vi "MTWIPbyPackage.vi"() -> ()   [LabVIEW 2012]
uses:
  <vilib>/Utility/NIReport.llb/NI_report.lvclass
  <vilib>/addons/database/Connection.llb/DB Tools Open Connec (Path).vi
  <vilib>/addons/database/Connection.llb/Conn Execute.vi
  <vilib>/addons/database/Recordset.llb/Rec Fetch Recordset Data (R).vi
  <vilib>/addons/database/Recordset.llb/Rec Destroy - Connection.vi
  <vilib>/Utility/NIReport.llb/Append Text Table to Report (wrap).vi
  <vilib>/addons/database/_DB Variant To Data/Database Variant To Data.xnode
  <vilib>/addons/database/NI_Database_API.lvlib
  <vilib>/Utility/NIReport.llb/Excel/NI_Excel.lvclass
  <vilib>/addons/_office/NI_ReportGenerationToolkit.lvlib
panel:
  out "recordset data 2":variant[][](array[variant])
  out "appended array 2":string[](array[string])
  out "error out 5":errorcluster
  in  "Report Template":path=path "O:/Monitor/Report/M100DailyWIP.xls"
  out "error out 2":errorcluster
  in  "Table Control":string[][](table)
  in  "Table Control 2":string[][](table)
  in  "Table Control 3":string[][](table)
  out "error out 4":errorcluster
  out "error out 3":errorcluster
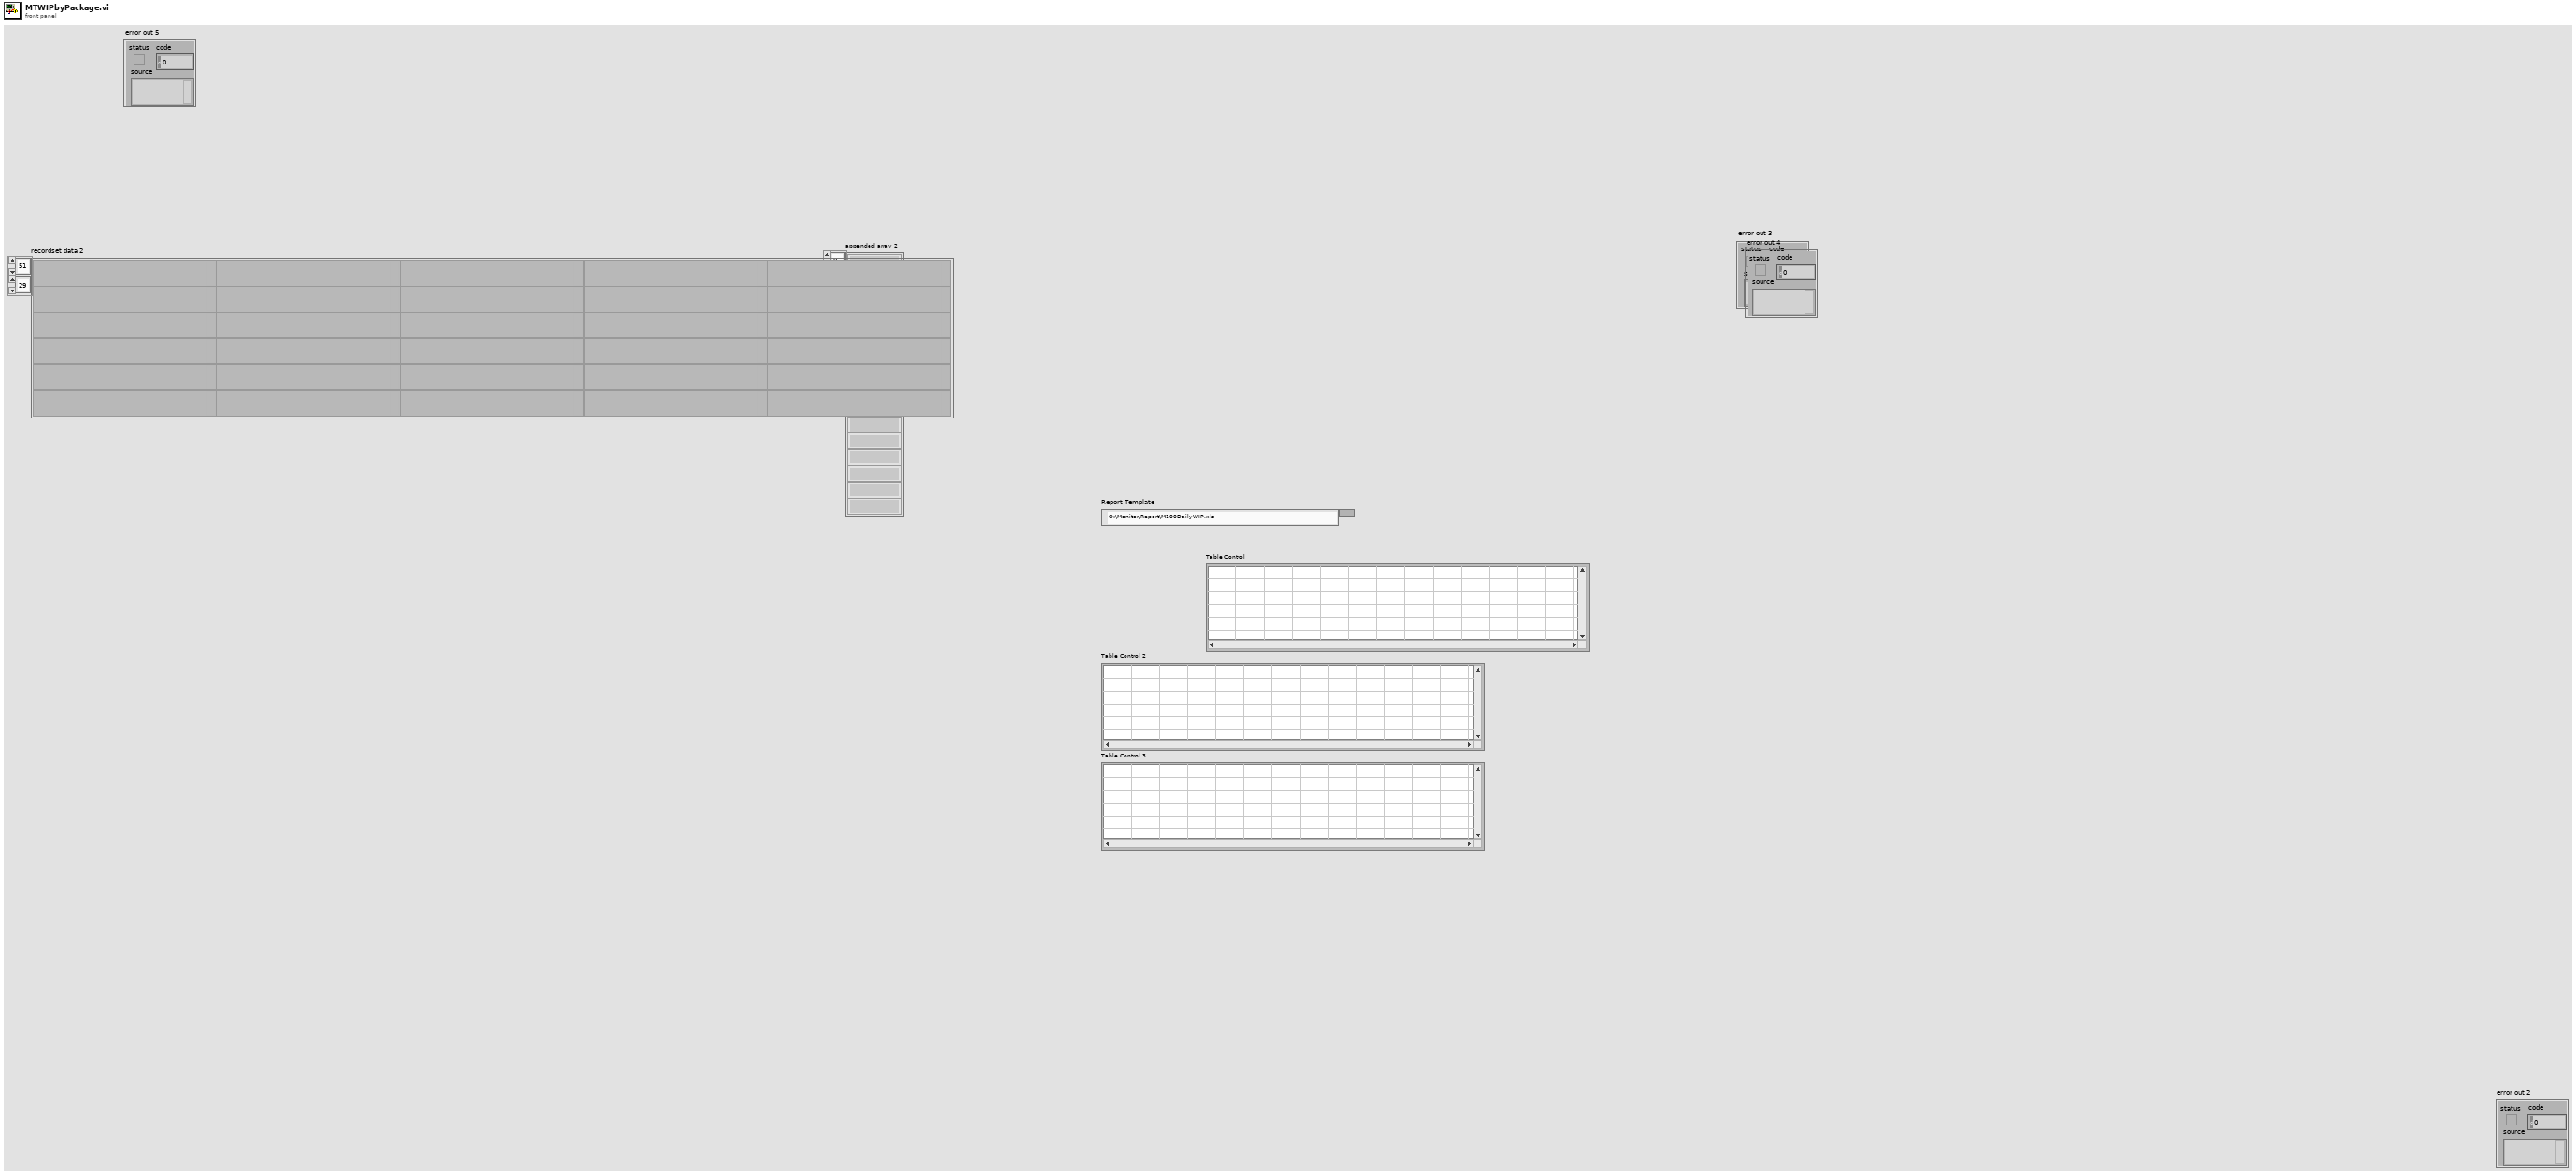
[diagram p1: front panel]
types:
  T1 = typedef "NI_Database_API.lvlib/Conn ObjectReference.ctl" = refnum<k1>
  T2 = typedef "NI_Database_API.lvlib/Rec ObjectReference.ctl" = refnum<k1>
  T3 = enum16{"Standard Report", "HTML", "Word", "Excel"}
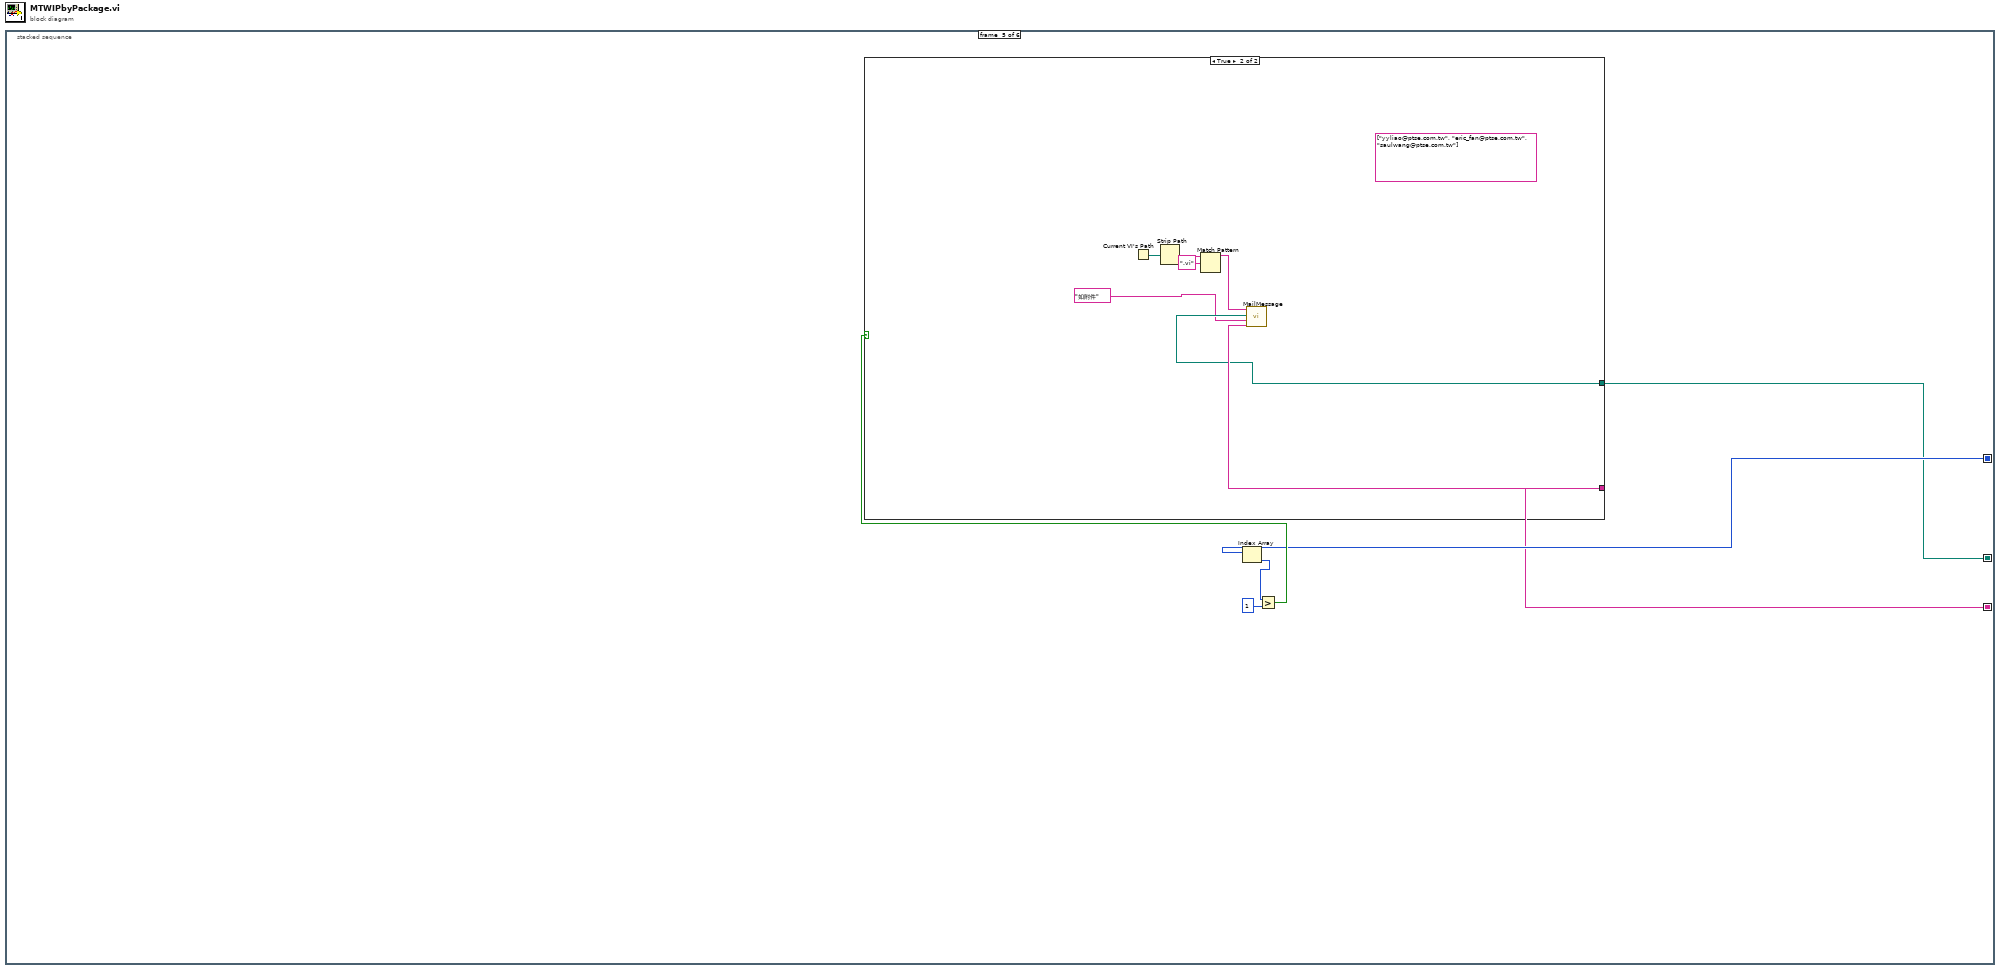
[diagram p0: block diagram]
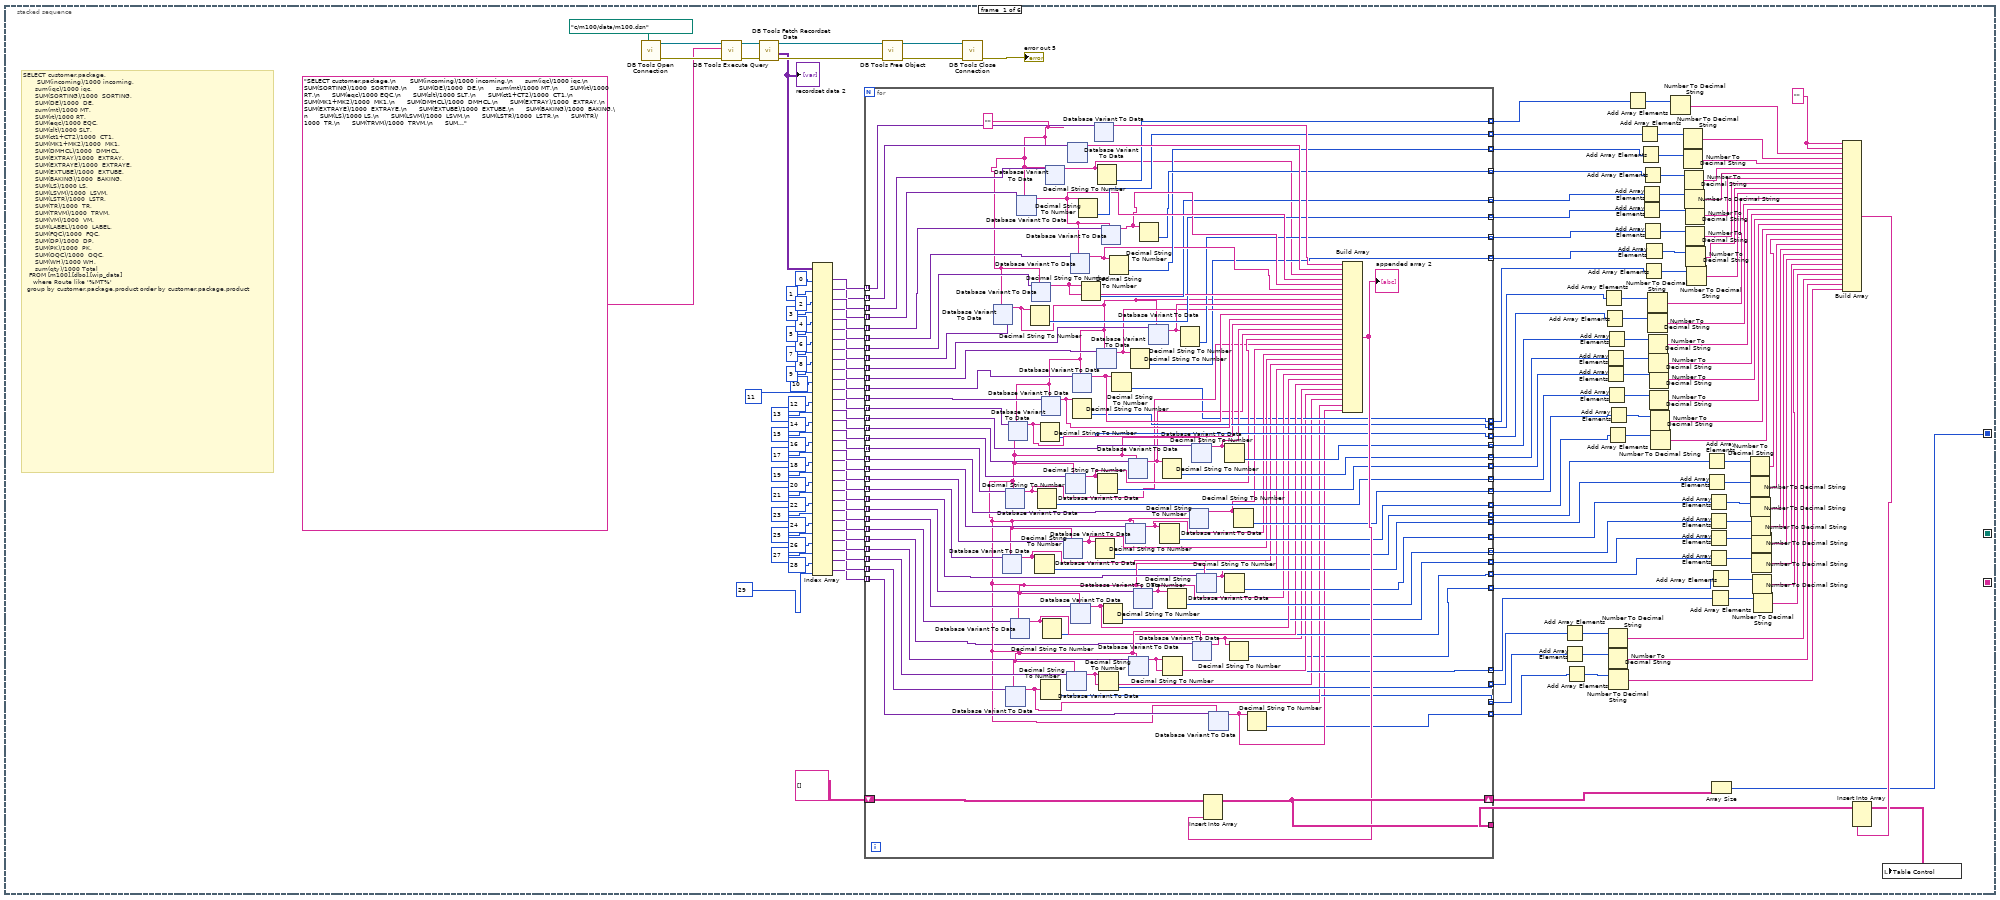
[diagram p2: hidden frame]
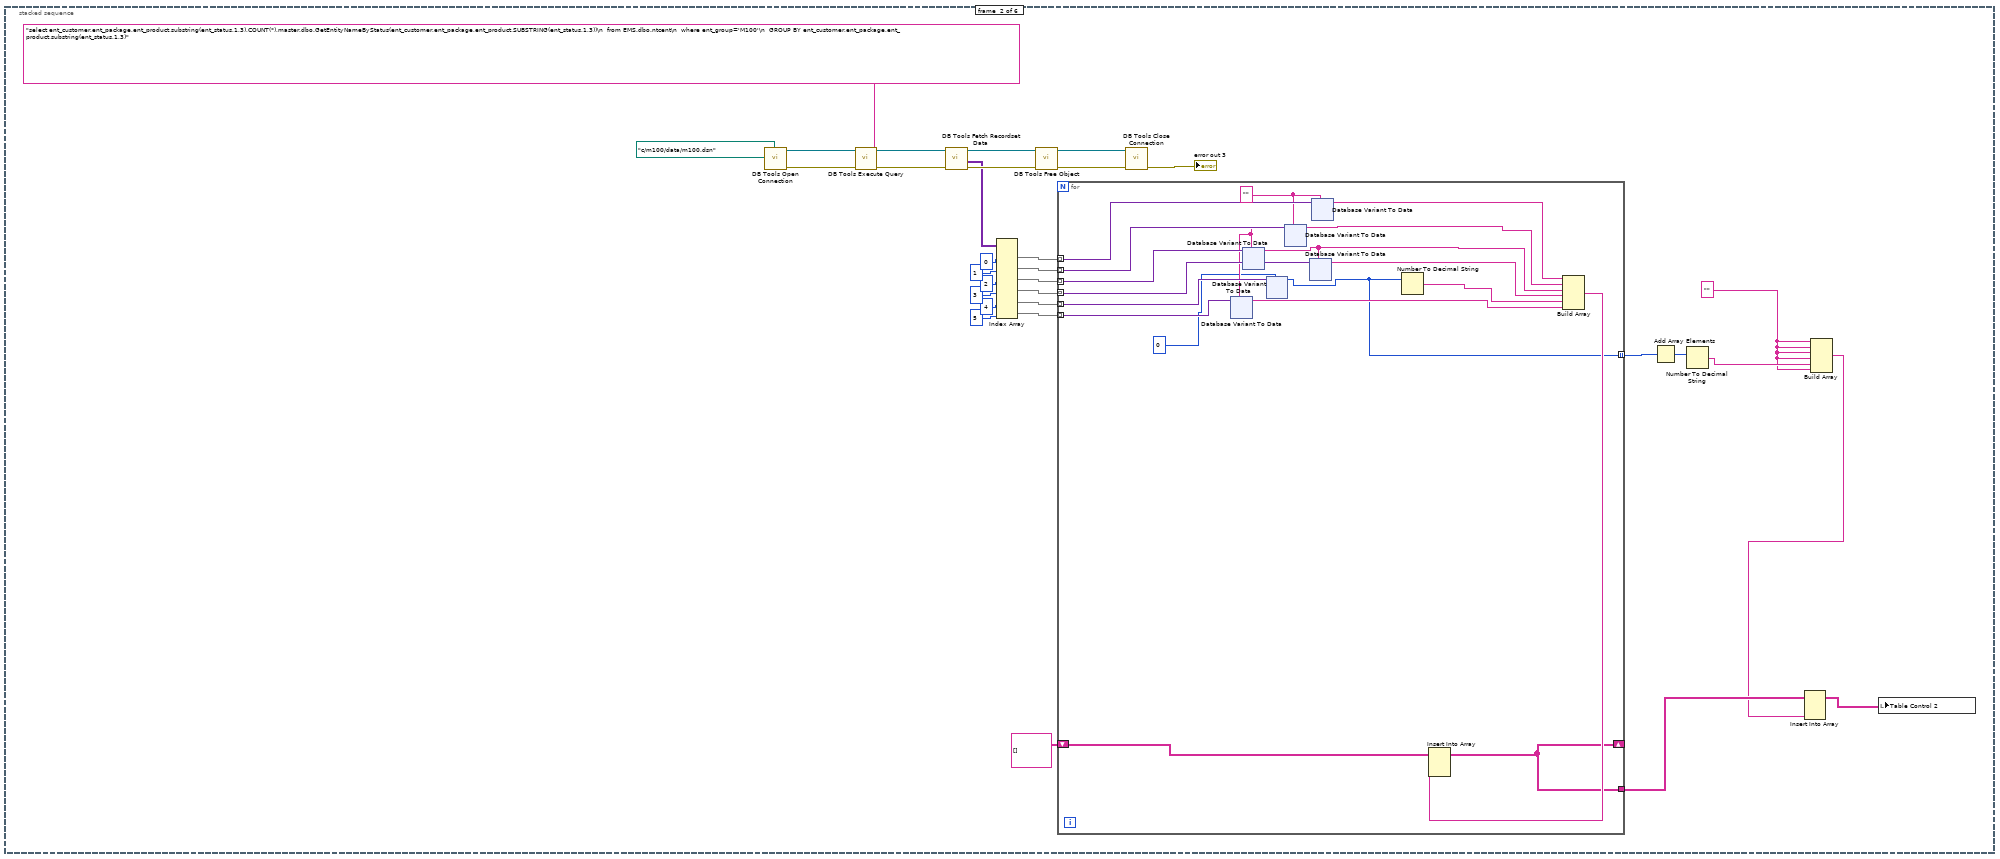
[diagram p3: hidden frame]
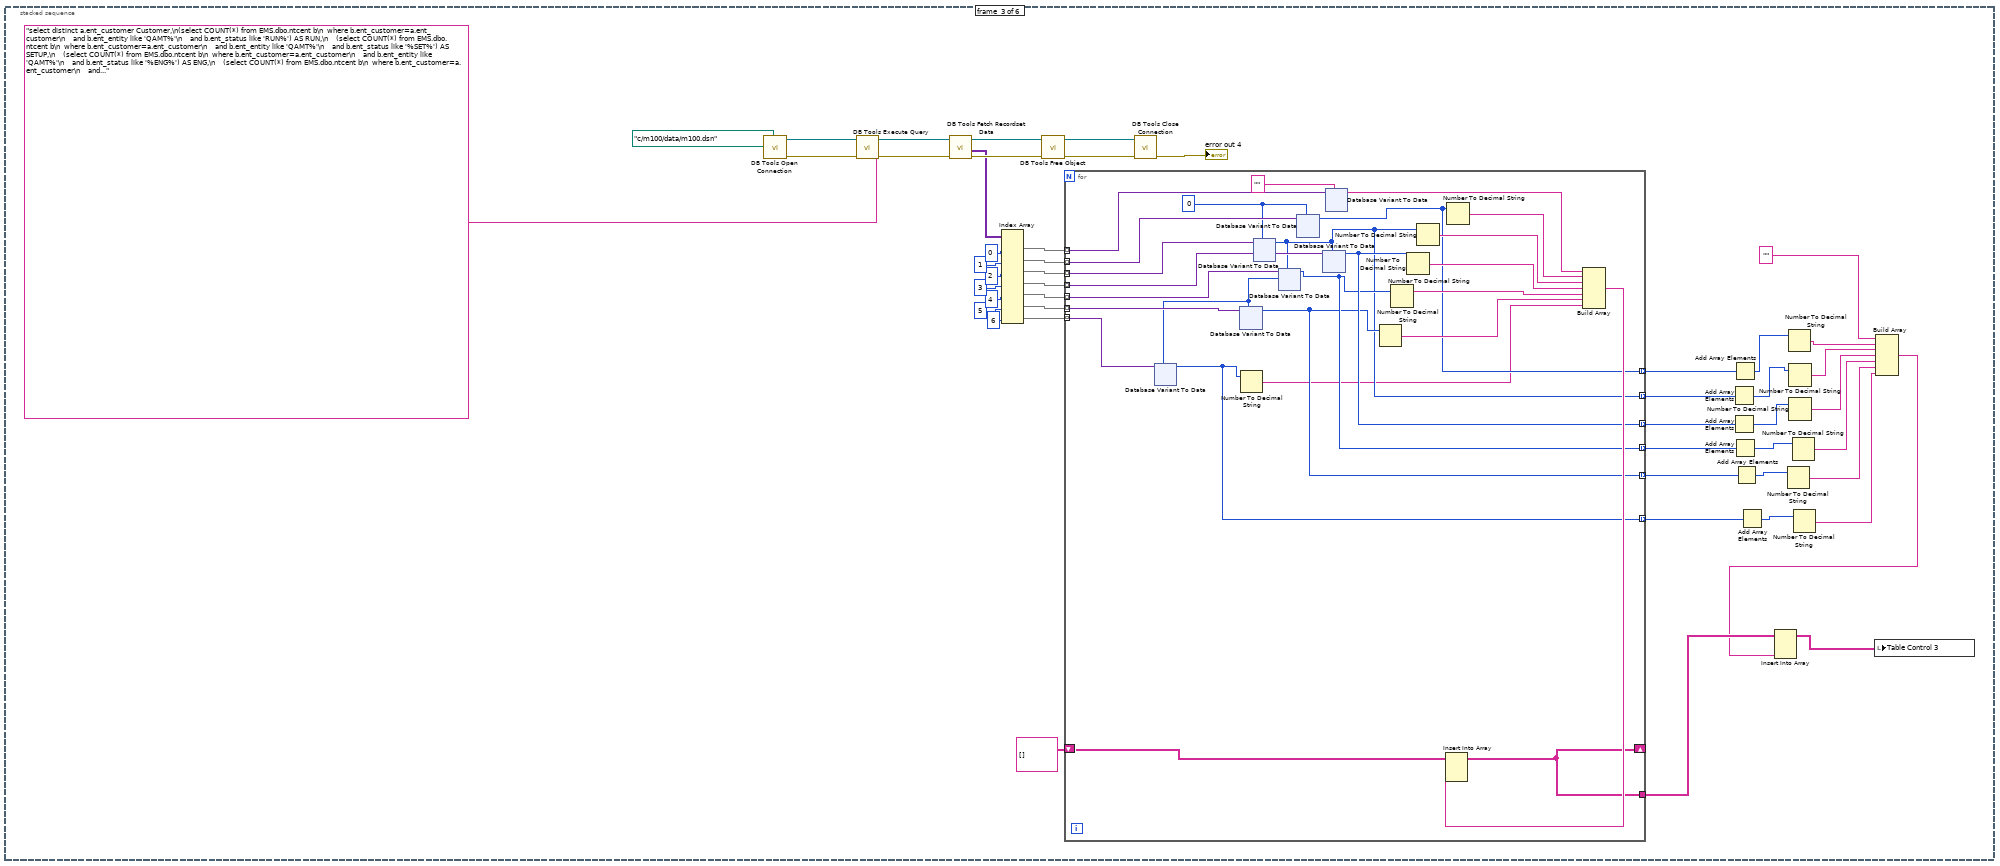
[diagram p4: hidden frame]
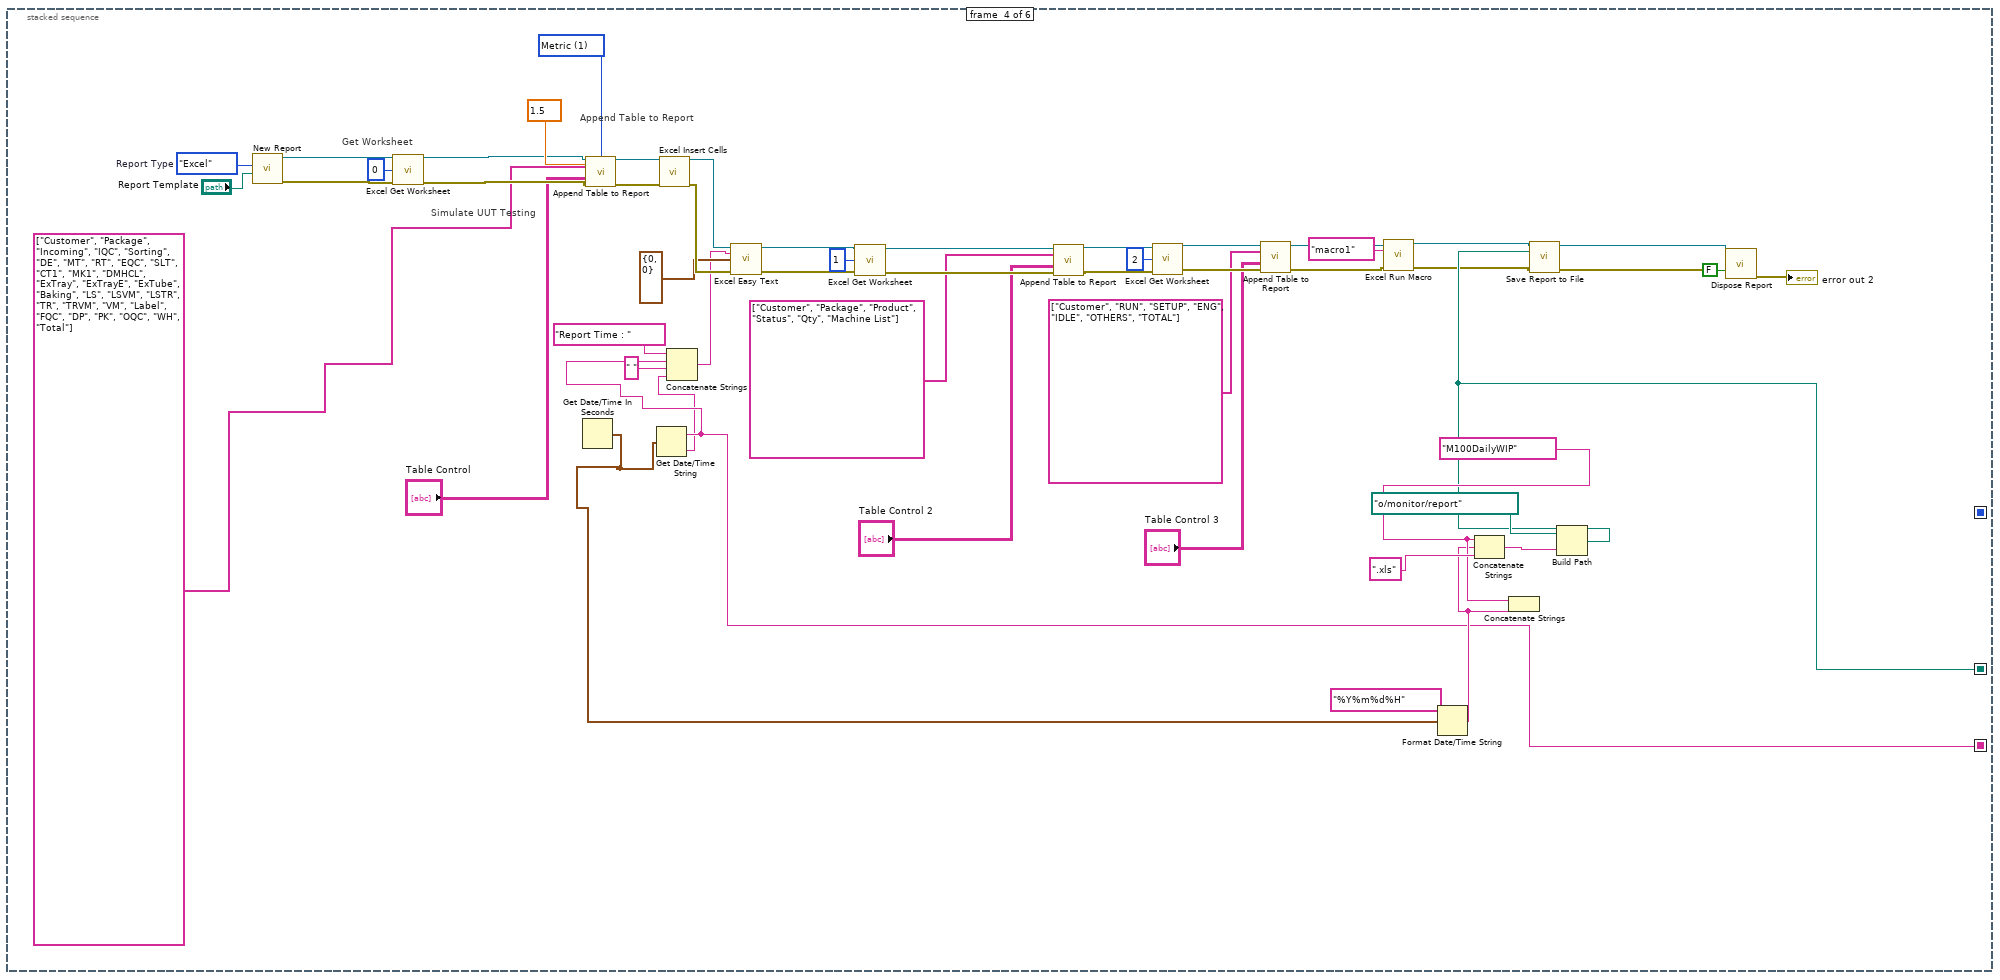
[diagram p5: hidden frame]
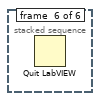
[diagram p7: hidden frame]
diagram:
  n1 = stacked-sequence {
    seq-local: [w2 _ _ _ _ _] -> [_ _ _ _ w1810 _]
    seq-local: [_ _ _ w1781 _ _] -> [_ _ _ _ w1809 _]
    seq-local: [_ _ _ w1758 _ _] -> [_ _ _ _ w1808 _]
    frame #0 {
      w4 = ""
      # "SELECT customer,package,\n       SUM(incoming)/1000 incoming,\n      sum(iqc)/1000 iqc,\n      SUM(SORTING)/1000  SORTING,\n      SUM(DE)/1000  DE,\n      sum(mt)/1000 MT,\n      SUM(rt)/1000 RT,\n      SUM(eqc)/1000 EQC,\n      SUM(slt)/1000 SLT,\n      SUM(ct1+CT2)/1000  CT1,\n      SUM(MK1+MK2)/1000  MK1,\n      SUM(DMHCL)/1000  DMHCL,\n      SUM(EXTRAY)/1000  EXTRAY,\n      SUM(EXTRAYE)/1000  EXTRAYE,\n      SUM(EXTUBE)/1000  EXTUBE,\n      SUM(BAKING)/1000  BAKING,\n      SUM(LS)/1000 LS,\n      SUM(LSVM)/1000  LSVM,\n      SUM(LSTR)/1000  LSTR,\n      SUM(TR)/1000  TR,\n      SUM(TRVM)/1000  TRVM,\n      SUM(VM)/1000  VM,\n      SUM(LABEL)/1000  LABEL,\n      SUM(FQC)/1000  FQC,\n      SUM(DP)/1000  DP,\n      SUM(PK)/1000  PK,\n      SUM(OQC)/1000  OQC,\n      SUM(WH)/1000 WH,\n      sum(qty)/1000 Total\n   FROM [m100].[dbo].[wip_data]\n     where Route like '%MT%'\n  group by customer,package,product order by customer,package,product"
      n2 = call-poly <vilib>:"DB Tools Open Connection.vi"("connection information"=path "c:/m100/data/m100.dsn") -> ("error out"=w158:errorcluster, "connection reference"=w162:T1)  [unwired: 7 in]
      n3 = call-poly <vilib>:"DB Tools Execute Query.vi"("error in (no error)"=w158, "SQL query"="SELECT customer,package,\n       SUM(incoming)/1000 incoming,\n      sum(iqc)/1000 iqc,\n      SUM(SORTING)/1000  SORTING,\n      SUM(DE)/1000  DE,\n      sum(mt)/1000 MT,\n      SUM(rt)/1000 RT,\n      SUM(eqc)/1000 EQC,\n      SUM(slt)/1000 SLT,\n      SUM(ct1+CT2)/1000  CT1,\n      SUM(MK1+MK2)/1000  MK1,\n      SUM(DMHCL)/1000  DMHCL,\n      SUM(EXTRAY)/1000  EXTRAY,\n      SUM(EXTRAYE)/1000  EXTRAYE,\n      SUM(EXTUBE)/1000  EXTUBE,\n      SUM(BAKING)/1000  BAKING,\n      SUM(LS)/1000 LS,\n      SUM(LSVM)/1000  LSVM,\n      SUM(LSTR)/1000  LSTR,\n      SUM(TR)/1000  TR,\n      SUM(TRVM)/1000  TRVM,\n      SUM(VM)/1000  VM,\n      SUM(LABEL)/1000  LABEL,\n      SUM(FQC)/1000  FQC,\n      SUM(DP)/1000  DP,\n      SUM(PK)/1000  PK,\n      SUM(OQC)/1000  OQC,\n      SUM(WH)/1000 WH,\n      sum(qty)/1000 Total\n   FROM [m100].[dbo].[wip_data]\n     where Route like '%MT%'\n  group by customer,package order by customer,package", "connection reference"=w162) -> ("error out"=w157:errorcluster, "recordset reference"=w161:T2)  [unwired: 5 in]
      n4 = call-poly <vilib>:"DB Tools Fetch Recordset Data.vi"("error in (no error)"=w157, "recordset reference"=w161) -> ("error out"=w156:errorcluster, "recordset data"=w126:variant[][], "recordset reference out"=w160:T2)  [unwired: 3 in]
      "recordset data 2" <- w126
      n5 = Index Array(array=w126, index (col) #1=0 ("index (row)"), index (col) #2=1 ("index (col)"), index (col) #3=2 ("disabled index (col)"), index (col) #4=3 ("index (col)"), index (col) #5=4 ("index (col)"), index (col) #6=5 ("index (col)"), index (col) #7=6 ("index (col)"), index (col) #8=7 ("index (col)"), index (col) #9=8 ("index (col)"), index (col) #10=9 ("index (col)"), index (col) #11=10 ("index (col)"), index (col) #12=11 ("index (col)"), index (col) #13=12 ("index (col)"), index (col) #14=13 ("index (col)"), index (col) #15=14 ("index (col)"), index (col) #16=15 ("index (col)"), index (col) #17=16 ("index (col)"), index (col) #18=17 ("index (col)"), index (col) #19=18 ("index (col)"), index (col) #20=19 ("index (col)"), index (col) #21=20 ("index (col)"), index (col) #22=21 ("index (col)"), index (col) #23=22 ("index (col)"), index (col) #24=23 ("index (col)"), index (col) #25=24 ("index (col)"), index (col) #26=25 ("index (col)"), index (col) #27=26 ("index (col)"), index (col) #28=27 ("index (col)"), index (col) #29=28 ("index (col)"), index (col) #30=29 ("index (col)")) -> (element #1=w130:variant[], element #2=w129:variant[], element #3=w143:variant[], element #4=w142:variant[], element #5=w141:variant[], element #6=w140:variant[], element #7=w139:variant[], element #8=w138:variant[], element #9=w137:variant[], element #10=w136:variant[], element #11=w135:variant[], element #12=w134:variant[], element #13=w103:variant[], element #14=w102:variant[], element #15=w101:variant[], element #16=w100:variant[], element #17=w99:variant[], element #18=w98:variant[], element #19=w97:variant[], element #20=w96:variant[], element #21=w95:variant[], element #22=w94:variant[], element #23=w93:variant[], element #24=w92:variant[], element #25=w91:variant[], element #26=w90:variant[], element #27=w89:variant[], element #28=w88:variant[], element #29=w87:variant[], element #30=w86:variant[])  [unwired: 30 in]
      n6 = for {
        tunnel: w143 -> [w249] mode=indexing
        tunnel: w142 -> [w248] mode=indexing
        tunnel: w141 -> [w247] mode=indexing
        tunnel: w140 -> [w246] mode=indexing
        tunnel: w139 -> [w245] mode=indexing
        tunnel: w138 -> [w244] mode=indexing
        tunnel: w137 -> [w243] mode=indexing
        tunnel: w136 -> [w242] mode=indexing
        tunnel: w135 -> [w241] mode=indexing
        tunnel: w134 -> [w240] mode=indexing
        tunnel: [w255] -> w122
        shift-right: [w255] -> w132
        shift-left: string[][] [] ("array") -> [w254]
        tunnel: w130 -> [w251] mode=indexing
        tunnel: w129 -> [w250] mode=indexing
        tunnel: w103 -> [w238] mode=indexing
        tunnel: w102 -> [w237] mode=indexing
        tunnel: w101 -> [w236] mode=indexing
        tunnel: w100 -> [w235] mode=indexing
        tunnel: w99 -> [w234] mode=indexing
        tunnel: w98 -> [w233] mode=indexing
        tunnel: w97 -> [w230] mode=indexing
        tunnel: w96 -> [w232] mode=indexing
        tunnel: w95 -> [w231] mode=indexing
        tunnel: w94 -> [w229] mode=indexing
        tunnel: w93 -> [w228] mode=indexing
        tunnel: w92 -> [w226] mode=indexing
        tunnel: w91 -> [w227] mode=indexing
        tunnel: w90 -> [w166] mode=indexing
        tunnel: w89 -> [w225] mode=indexing
        tunnel: w88 -> [w224] mode=indexing
        tunnel: w87 -> [w223] mode=indexing
        tunnel: w86 -> [w222] mode=indexing
        tunnel: [w214] -> w6 mode=indexing
        tunnel: [w217] -> w60 mode=indexing
        tunnel: [w218] -> w59 mode=indexing
        tunnel: [w213] -> w58 mode=indexing
        tunnel: [w211] -> w57 mode=indexing
        tunnel: [w209] -> w56 mode=indexing
        tunnel: [w207] -> w55 mode=indexing
        tunnel: [w175] -> w54 mode=indexing
        tunnel: [w203] -> w53 mode=indexing
        tunnel: [w201] -> w52 mode=indexing
        tunnel: [w199] -> w51 mode=indexing
        tunnel: [w197] -> w50 mode=indexing
        tunnel: [w195] -> w49 mode=indexing
        tunnel: [w193] -> w48 mode=indexing
        tunnel: [w192] -> w47 mode=indexing
        tunnel: [w189] -> w46 mode=indexing
        tunnel: [w187] -> w45 mode=indexing
        tunnel: [w185] -> w44 mode=indexing
        tunnel: [w183] -> w43 mode=indexing
        tunnel: [w181] -> w42 mode=indexing
        tunnel: [w179] -> w41 mode=indexing
        tunnel: [w177] -> w40 mode=indexing
        tunnel: [w164] -> w39 mode=indexing
        tunnel: [w173] -> w38 mode=indexing
        tunnel: [w171] -> w37 mode=indexing
        tunnel: [w169] -> w36 mode=indexing
        tunnel: [w167] -> w35 mode=indexing
        tunnel: [w221] -> w5 mode=indexing
        w215 = ""
        n7 = xnode "Database Variant To Data"("database variant"=w244, "type"=w215) -> ("data"=w206:string)  [unwired: 1 in, 1 out]
        n8 = xnode "Database Variant To Data"("database variant"=w238, "type"=w206) -> ("data"=w202:string)  [unwired: 1 in, 1 out]
        n9 = xnode "Database Variant To Data"("database variant"=w231, "type"=w202) -> ("data"=w186:string)  [unwired: 1 in, 1 out]
        n10 = xnode "Database Variant To Data"("database variant"=w234, "type"=w202) -> ("data"=w194:string)  [unwired: 1 in, 1 out]
        n11 = xnode "Database Variant To Data"("database variant"=w223, "type"=w202) -> ("data"=w170:string)  [unwired: 1 in, 1 out]
        n12 = xnode "Database Variant To Data"("database variant"=w227, "type"=w202) -> ("data"=w178:string)  [unwired: 1 in, 1 out]
        n13 = xnode "Database Variant To Data"("database variant"=w248, "type"=w215) -> ("data"=w220:string)  [unwired: 1 in, 1 out]
        n14 = Decimal String To Number(string=w206) -> (number=w211:i32)  [unwired: 2 in, 1 out]
        n15 = xnode "Database Variant To Data"("database variant"=w245, "type"=w215) -> ("data"=w212:string)  [unwired: 1 in, 1 out]
        n16 = Decimal String To Number(string=w186) -> (number=w185:i32)  [unwired: 2 in, 1 out]
        n17 = Decimal String To Number(string=w194) -> (number=w193:i32)  [unwired: 2 in, 1 out]
        n18 = Decimal String To Number(string=w202) -> (number=w201:i32)  [unwired: 2 in, 1 out]
        n19 = Decimal String To Number(string=w170) -> (number=w169:i32)  [unwired: 2 in, 1 out]
        n20 = xnode "Database Variant To Data"("database variant"=w240, "type"=w206) -> ("data"=w204:string)  [unwired: 1 in, 1 out]
        n21 = Decimal String To Number(string=w178) -> (number=w177:i32)  [unwired: 2 in, 1 out]
        n22 = xnode "Database Variant To Data"("database variant"=w249, "type"=w215) -> ("data"=w165:string)  [unwired: 1 in, 1 out]
        n23 = xnode "Database Variant To Data"("database variant"=w232, "type"=w202) -> ("data"=w188:string)  [unwired: 1 in, 1 out]
        n24 = xnode "Database Variant To Data"("database variant"=w235, "type"=w202) -> ("data"=w196:string)  [unwired: 1 in, 1 out]
        n25 = xnode "Database Variant To Data"("database variant"=w224, "type"=w202) -> ("data"=w172:string)  [unwired: 1 in, 1 out]
        n26 = xnode "Database Variant To Data"("database variant"=w250, "type"=w215) -> ("data"=w252:string)  [unwired: 1 in, 1 out]
        n27 = xnode "Database Variant To Data"("database variant"=w246, "type"=w220) -> ("data"=w216:string)  [unwired: 1 in, 1 out]
        n28 = xnode "Database Variant To Data"("database variant"=w226, "type"=w202) -> ("data"=w180:string)  [unwired: 1 in, 1 out]
        n29 = xnode "Database Variant To Data"("database variant"=w241, "type"=w206) -> ("data"=w205:string)  [unwired: 1 in, 1 out]
        n30 = Decimal String To Number(string=w204) -> (number=w203:i32)  [unwired: 2 in, 1 out]
        n31 = Decimal String To Number(string=w220) -> (number=w221:i32)  [unwired: 2 in, 1 out]
        n32 = Decimal String To Number(string=w212) -> (number=w213:i32)  [unwired: 2 in, 1 out]
        n33 = xnode "Database Variant To Data"("database variant"=w251, "type"=w215) -> ("data"=w253:string)  [unwired: 1 in, 1 out]
        n34 = Decimal String To Number(string=w188) -> (number=w187:i32)  [unwired: 2 in, 1 out]
        n35 = xnode "Database Variant To Data"("database variant"=w242, "type"=w206) -> ("data"=w208:string)  [unwired: 1 in, 1 out]
        n36 = Decimal String To Number(string=w165) -> (number=w214:i32)  [unwired: 2 in, 1 out]
        n37 = Decimal String To Number(string=w196) -> (number=w195:i32)  [unwired: 2 in, 1 out]
        n38 = Decimal String To Number(string=w172) -> (number=w171:i32)  [unwired: 2 in, 1 out]
        n39 = xnode "Database Variant To Data"("database variant"=w247, "type"=w220) -> ("data"=w219:string)  [unwired: 1 in, 1 out]
        n40 = Decimal String To Number(string=w180) -> (number=w179:i32)  [unwired: 2 in, 1 out]
        n41 = Decimal String To Number(string=w216) -> (number=w217:i32)  [unwired: 2 in, 1 out]
        n42 = Decimal String To Number(string=w205) -> (number=w175:i32)  [unwired: 2 in, 1 out]
        n43 = xnode "Database Variant To Data"("database variant"=w230, "type"=w202) -> ("data"=w190:string)  [unwired: 1 in, 1 out]
        n44 = xnode "Database Variant To Data"("database variant"=w236, "type"=w202) -> ("data"=w198:string)  [unwired: 1 in, 1 out]
        n45 = xnode "Database Variant To Data"("database variant"=w225, "type"=w202) -> ("data"=w174:string)  [unwired: 1 in, 1 out]
        n46 = Decimal String To Number(string=w208) -> (number=w207:i32)  [unwired: 2 in, 1 out]
        n47 = xnode "Database Variant To Data"("database variant"=w228, "type"=w202) -> ("data"=w182:string)  [unwired: 1 in, 1 out]
        n48 = Decimal String To Number(string=w219) -> (number=w218:i32)  [unwired: 2 in, 1 out]
        n49 = xnode "Database Variant To Data"("database variant"=w243, "type"=w206) -> ("data"=w210:string)  [unwired: 1 in, 1 out]
        n50 = Decimal String To Number(string=w190) -> (number=w189:i32)  [unwired: 2 in, 1 out]
        n51 = Decimal String To Number(string=w198) -> (number=w197:i32)  [unwired: 2 in, 1 out]
        n52 = Decimal String To Number(string=w174) -> (number=w173:i32)  [unwired: 2 in, 1 out]
        n53 = Decimal String To Number(string=w182) -> (number=w181:i32)  [unwired: 2 in, 1 out]
        n54 = Decimal String To Number(string=w210) -> (number=w209:i32)  [unwired: 2 in, 1 out]
        n55 = xnode "Database Variant To Data"("database variant"=w233, "type"=w202) -> ("data"=w191:string)  [unwired: 1 in, 1 out]
        n56 = xnode "Database Variant To Data"("database variant"=w237, "type"=w202) -> ("data"=w200:string)  [unwired: 1 in, 1 out]
        n57 = xnode "Database Variant To Data"("database variant"=w166, "type"=w202) -> ("data"=w176:string)  [unwired: 1 in, 1 out]
        n58 = xnode "Database Variant To Data"("database variant"=w229, "type"=w202) -> ("data"=w184:string)  [unwired: 1 in, 1 out]
        n59 = xnode "Database Variant To Data"("database variant"=w222, "type"=w202) -> ("data"=w168:string)  [unwired: 1 in, 1 out]
        n60 = Decimal String To Number(string=w200) -> (number=w199:i32)  [unwired: 2 in, 1 out]
        n61 = Decimal String To Number(string=w184) -> (number=w183:i32)  [unwired: 2 in, 1 out]
        n62 = Decimal String To Number(string=w176) -> (number=w164:i32)  [unwired: 2 in, 1 out]
        n63 = Decimal String To Number(string=w191) -> (number=w192:i32)  [unwired: 2 in, 1 out]
        n64 = Decimal String To Number(string=w168) -> (number=w167:i32)  [unwired: 2 in, 1 out]
        n65 = Build Array(w253, w252, w165, w220, w219, w216, w212, w206, w210, w208, w205, w204, w202, w200, w198, w196, w194, w191, w190, w188, w186, w184, w182, w180, w178, w176, w174, w172, w170, w168) -> (w239:string[])
        "appended array 2" <- w239
        n66 = Insert Into Array(array=w254, new element=w239) -> (w255:string[][])  [unwired: 2 in]
      }
      n67 = call-poly <vilib>:"DB Tools Free Object.vi"("error in (no error)"=w156, "recordset reference"=w160) -> ("error out"=w155:errorcluster, "connection reference"=w159:T1)  [unwired: 8 in]
      n68 = call <vilib>:"DB Tools Close Connection.vi"("error in (no error)"=w155, "connection reference"=w159) -> ("error out"=→"error out 5":errorcluster)  [unwired: 5 in]
      n69 = Add Array Elements(numeric array=w37) -> (sum=w63:i32)
      n70 = Add Array Elements(numeric array=w36) -> (sum=w62:i32)
      n71 = Add Array Elements(numeric array=w35) -> (sum=w61:i32)
      n72 = Add Array Elements(numeric array=w53) -> (sum=w79:i32)
      n73 = Add Array Elements(numeric array=w52) -> (sum=w78:i32)
      n74 = Add Array Elements(numeric array=w50) -> (sum=w76:i32)
      n75 = Add Array Elements(numeric array=w49) -> (sum=w75:i32)
      n76 = Add Array Elements(numeric array=w51) -> (sum=w77:i32)
      n77 = Add Array Elements(numeric array=w48) -> (sum=w74:i32)
      n78 = Add Array Elements(numeric array=w46) -> (sum=w72:i32)
      n79 = Number To Decimal String(number=w63) -> (decimal integer string=w10:string)  [unwired: 1 in]
      n80 = Number To Decimal String(number=w62) -> (decimal integer string=w9:string)  [unwired: 1 in]
      n81 = Add Array Elements(numeric array=w47) -> (sum=w73:i32)
      n82 = Number To Decimal String(number=w61) -> (decimal integer string=w8:string)  [unwired: 1 in]
      n83 = Add Array Elements(numeric array=w6) -> (sum=w7:i32)
      n84 = Add Array Elements(numeric array=w5) -> (sum=w125:i32)
      n85 = Add Array Elements(numeric array=w60) -> (sum=w124:i32)
      n86 = Add Array Elements(numeric array=w58) -> (sum=w84:i32)
      n87 = Add Array Elements(numeric array=w57) -> (sum=w83:i32)
      n88 = Add Array Elements(numeric array=w59) -> (sum=w85:i32)
      n89 = Add Array Elements(numeric array=w56) -> (sum=w82:i32)
      n90 = Add Array Elements(numeric array=w54) -> (sum=w80:i32)
      n91 = Add Array Elements(numeric array=w55) -> (sum=w81:i32)
      n92 = Number To Decimal String(number=w79) -> (decimal integer string=w26:string)  [unwired: 1 in]
      n93 = Number To Decimal String(number=w78) -> (decimal integer string=w25:string)  [unwired: 1 in]
      n94 = Number To Decimal String(number=w77) -> (decimal integer string=w24:string)  [unwired: 1 in]
      n95 = Number To Decimal String(number=w76) -> (decimal integer string=w23:string)  [unwired: 1 in]
      n96 = Number To Decimal String(number=w75) -> (decimal integer string=w22:string)  [unwired: 1 in]
      n97 = Number To Decimal String(number=w74) -> (decimal integer string=w21:string)  [unwired: 1 in]
      n98 = Number To Decimal String(number=w73) -> (decimal integer string=w20:string)  [unwired: 1 in]
      n99 = Number To Decimal String(number=w72) -> (decimal integer string=w19:string)  [unwired: 1 in]
      n100 = Number To Decimal String(number=w7) -> (decimal integer string=w3:string)  [unwired: 1 in]
      n101 = Number To Decimal String(number=w125) -> (decimal integer string=w34:string)  [unwired: 1 in]
      n102 = Number To Decimal String(number=w124) -> (decimal integer string=w33:string)  [unwired: 1 in]
      n103 = Number To Decimal String(number=w85) -> (decimal integer string=w32:string)  [unwired: 1 in]
      n104 = Number To Decimal String(number=w84) -> (decimal integer string=w31:string)  [unwired: 1 in]
      n105 = Number To Decimal String(number=w83) -> (decimal integer string=w30:string)  [unwired: 1 in]
      n106 = Number To Decimal String(number=w82) -> (decimal integer string=w29:string)  [unwired: 1 in]
      n107 = Number To Decimal String(number=w81) -> (decimal integer string=w28:string)  [unwired: 1 in]
      n108 = Number To Decimal String(number=w80) -> (decimal integer string=w27:string)  [unwired: 1 in]
      n109 = Add Array Elements(numeric array=w45) -> (sum=w71:i32)
      n110 = Add Array Elements(numeric array=w44) -> (sum=w70:i32)
      n111 = Add Array Elements(numeric array=w42) -> (sum=w68:i32)
      n112 = Add Array Elements(numeric array=w41) -> (sum=w67:i32)
      n113 = Add Array Elements(numeric array=w43) -> (sum=w69:i32)
      n114 = Add Array Elements(numeric array=w40) -> (sum=w66:i32)
      n115 = Add Array Elements(numeric array=w38) -> (sum=w64:i32)
      n116 = Add Array Elements(numeric array=w39) -> (sum=w65:i32)
      n117 = Array Size(array=w132) -> (size(s)=w2:i32[])
      n118 = Number To Decimal String(number=w71) -> (decimal integer string=w18:string)  [unwired: 1 in]
      n119 = Number To Decimal String(number=w70) -> (decimal integer string=w17:string)  [unwired: 1 in]
      n120 = Number To Decimal String(number=w69) -> (decimal integer string=w16:string)  [unwired: 1 in]
      n121 = Number To Decimal String(number=w68) -> (decimal integer string=w15:string)  [unwired: 1 in]
      n122 = Number To Decimal String(number=w67) -> (decimal integer string=w14:string)  [unwired: 1 in]
      n123 = Number To Decimal String(number=w66) -> (decimal integer string=w13:string)  [unwired: 1 in]
      n124 = Number To Decimal String(number=w65) -> (decimal integer string=w12:string)  [unwired: 1 in]
      n125 = Number To Decimal String(number=w64) -> (decimal integer string=w11:string)  [unwired: 1 in]
      n126 = Build Array(w4, w4, w3, w34, w33, w32, w31, w30, w29, w28, w27, w26, w25, w24, w23, w22, w21, w20, w19, w18, w17, w16, w15, w14, w13, w12, w11, w10, w9, w8) -> (w123:string[])
      n127 = Insert Into Array(array=w122, new element=w123) -> (w1:string[][])  [unwired: 2 in]
      n128 = local write "Table Control"(w1) -> ()
    }
    frame #1 {
      w1217 = ""
      n129 = call-poly <vilib>:"DB Tools Open Connection.vi"("connection information"=path "c:/m100/data/m100.dsn") -> ("error out"=w1242:errorcluster, "connection reference"=w1246:T1)  [unwired: 7 in]
      n130 = call-poly <vilib>:"DB Tools Execute Query.vi"("error in (no error)"=w1242, "SQL query"="select ent_customer,ent_package,ent_product,substring(ent_status,1,3),COUNT(*),master.dbo.GetEntityNameByStatus(ent_customer,ent_package,ent_product,SUBSTRING(ent_status,1,3))\n  from EMS.dbo.ntcent\n  where ent_group='M100'\n  GROUP BY ent_customer,ent_package,ent_product,substring(ent_status,1,3)", "connection reference"=w1246) -> ("error out"=w1241:errorcluster, "recordset reference"=w1245:T2)  [unwired: 5 in]
      n131 = call-poly <vilib>:"DB Tools Fetch Recordset Data.vi"("error in (no error)"=w1241, "recordset reference"=w1245) -> ("error out"=w1240:errorcluster, "recordset data"=w1224:variant[][], "recordset reference out"=w1244:T2)  [unwired: 3 in]
      n132 = Index Array(array=w1224, index (col) #1=0 ("disabled index (col)"), index (col) #2=1 ("index (col)"), index (col) #3=2 ("index (col)"), index (col) #4=3 ("index (col)"), index (col) #5=4 ("index (col)"), index (col) #6=5 ("index (col)")) -> (element #1=w1231:variant[], element #2=w1230:variant[], element #3=w1229:variant[], element #4=w1228:variant[], element #5=w1227:variant[], element #6=w1226:variant[])  [unwired: 6 in]
      n133 = call-poly <vilib>:"DB Tools Free Object.vi"("error in (no error)"=w1240, "recordset reference"=w1244) -> ("error out"=w1239:errorcluster, "connection reference"=w1243:T1)  [unwired: 8 in]
      n134 = for {
        tunnel: w1231 -> [w1265] mode=indexing
        tunnel: w1230 -> [w1264] mode=indexing
        tunnel: w1229 -> [w1263] mode=indexing
        tunnel: w1228 -> [w1262] mode=indexing
        tunnel: w1227 -> [w1261] mode=indexing
        tunnel: w1226 -> [w1260] mode=indexing
        tunnel: [w1257] -> w1220
        shift-right: [w1257] -> _
        shift-left: string[][] [] -> [w1256]
        tunnel: [w1248] -> w1222 mode=indexing
        w1251 = ""
        n135 = xnode "Database Variant To Data"("database variant"=w1260, "type"=w1251) -> ("data"=w1252:string)  [unwired: 1 in, 1 out]
        n136 = xnode "Database Variant To Data"("database variant"=w1263, "type"=w1251) -> ("data"=w1253:string)  [unwired: 1 in, 1 out]
        n137 = xnode "Database Variant To Data"("database variant"=w1261, "type"=0) -> ("data"=w1248:i32)  [unwired: 1 in, 1 out]
        n138 = xnode "Database Variant To Data"("database variant"=w1264, "type"=w1251) -> ("data"=w1255:string)  [unwired: 1 in, 1 out]
        n139 = xnode "Database Variant To Data"("database variant"=w1262, "type"=w1253) -> ("data"=w1254:string)  [unwired: 1 in, 1 out]
        n140 = xnode "Database Variant To Data"("database variant"=w1265, "type"=w1251) -> ("data"=w1259:string)  [unwired: 1 in, 1 out]
        n141 = Number To Decimal String(number=w1248) -> (decimal integer string=w1249:string)  [unwired: 1 in]
        n142 = Build Array(w1259, w1255, w1253, w1254, w1249, w1252) -> (w1258:string[])
        n143 = Insert Into Array(array=w1256, new element=w1258) -> (w1257:string[][])  [unwired: 2 in]
      }
      n144 = call <vilib>:"DB Tools Close Connection.vi"("error in (no error)"=w1239, "connection reference"=w1243) -> ("error out"=→"error out 3":errorcluster)  [unwired: 5 in]
      n145 = Add Array Elements(numeric array=w1222) -> (sum=w1221:i32)
      n146 = Number To Decimal String(number=w1221) -> (decimal integer string=w1218:string)  [unwired: 1 in]
      n147 = Build Array(w1217, w1217, w1217, w1217, w1218, w1217) -> (w1216:string[])
      n148 = Insert Into Array(array=w1220, new element=w1216) -> (w1219:string[][])  [unwired: 2 in]
      n149 = local write "Table Control 2"(w1219) -> ()
    }
    frame #2 {
      n150 = call-poly <vilib>:"DB Tools Open Connection.vi"("connection information"=path "c:/m100/data/m100.dsn") -> ("error out"=w1501:errorcluster, "connection reference"=w1505:T1)  [unwired: 7 in]
      n151 = call-poly <vilib>:"DB Tools Execute Query.vi"("error in (no error)"=w1501, "SQL query"="select distinct a.ent_customer Customer,\n(select COUNT(*) from EMS.dbo.ntcent b\n  where b.ent_customer=a.ent_customer\n    and b.ent_entity like 'QAMT%'\n    and b.ent_status like 'RUN%') AS RUN,\n    (select COUNT(*) from EMS.dbo.ntcent b\n  where b.ent_customer=a.ent_customer\n    and b.ent_entity like 'QAMT%'\n    and b.ent_status like '%SET%') AS SETUP,\n    (select COUNT(*) from EMS.dbo.ntcent b\n  where b.ent_customer=a.ent_customer\n    and b.ent_entity like 'QAMT%'\n    and b.ent_status like '%ENG%') AS ENG,\n    (select COUNT(*) from EMS.dbo.ntcent b\n  where b.ent_customer=a.ent_customer\n    and b.ent_entity like 'QAMT%'\n    and b.ent_status like '%IDLE%') AS IDLE,\n    (select COUNT(*) from EMS.dbo.ntcent b\n  where b.ent_customer=a.ent_customer\n    and b.ent_entity like 'QAMT%'\n    and SUBSTRING(b.ent_status,1,3) NOT IN ('RUN','SET','ENG','IDL')) AS OTHERS,\n    (select COUNT(*) from EMS.dbo.ntcent b\n  where b.ent_customer=a.ent_customer\n    and b.ent_entity like 'QAMT%'\n    ) AS TOTAL\n    FROM EMS.dbo.ntcent a\n    where a.ent_entity like 'QAMT%'", "connection reference"=w1505) -> ("error out"=w1500:errorcluster, "recordset reference"=w1504:T2)  [unwired: 5 in]
      n152 = call-poly <vilib>:"DB Tools Fetch Recordset Data.vi"("error in (no error)"=w1500, "recordset reference"=w1504) -> ("error out"=w1499:errorcluster, "recordset data"=w1483:variant[][], "recordset reference out"=w1503:T2)  [unwired: 3 in]
      n153 = Index Array(array=w1483, index (col) #1=0 ("disabled index (col)"), index (col) #2=1 ("index (col)"), index (col) #3=2 ("index (col)"), index (col) #4=3 ("index (col)"), index (col) #5=4 ("index (col)"), index (col) #6=5 ("index (col)"), index (col) #7=6 ("index (col)")) -> (element #1=w1490:variant[], element #2=w1489:variant[], element #3=w1488:variant[], element #4=w1487:variant[], element #5=w1486:variant[], element #6=w1485:variant[], element #7=w1461:variant[])  [unwired: 7 in]
      n154 = call-poly <vilib>:"DB Tools Free Object.vi"("error in (no error)"=w1499, "recordset reference"=w1503) -> ("error out"=w1498:errorcluster, "connection reference"=w1502:T1)  [unwired: 8 in]
      n155 = for {
        tunnel: w1490 -> [w1531] mode=indexing
        tunnel: w1489 -> [w1530] mode=indexing
        tunnel: w1488 -> [w1529] mode=indexing
        tunnel: w1487 -> [w1528] mode=indexing
        tunnel: w1486 -> [w1527] mode=indexing
        tunnel: w1485 -> [w1526] mode=indexing
        tunnel: [w1523] -> w1464
        shift-right: [w1523] -> _
        shift-left: string[][] [] -> [w1522]
        tunnel: [w1514] -> w1481 mode=indexing
        tunnel: [w1509] -> w1480 mode=indexing
        tunnel: [w1513] -> w1479 mode=indexing
        tunnel: [w1512] -> w1478 mode=indexing
        tunnel: [w1511] -> w1477 mode=indexing
        tunnel: w1461 -> [w1510] mode=indexing
        tunnel: [w1507] -> w1459 mode=indexing
        w1520 = 0
        n156 = xnode "Database Variant To Data"("database variant"=w1529, "type"=w1520) -> ("data"=w1509:i32)  [unwired: 1 in, 1 out]
        n157 = xnode "Database Variant To Data"("database variant"=w1510, "type"=w1509) -> ("data"=w1507:i32)  [unwired: 1 in, 1 out]
        n158 = xnode "Database Variant To Data"("database variant"=w1526, "type"=w1509) -> ("data"=w1511:i32)  [unwired: 1 in, 1 out]
        n159 = Number To Decimal String(number=w1507) -> (decimal integer string=w1508:string)  [unwired: 1 in]
        n160 = xnode "Database Variant To Data"("database variant"=w1527, "type"=w1509) -> ("data"=w1512:i32)  [unwired: 1 in, 1 out]
        n161 = xnode "Database Variant To Data"("database variant"=w1530, "type"=w1520) -> ("data"=w1514:i32)  [unwired: 1 in, 1 out]
        n162 = xnode "Database Variant To Data"("database variant"=w1528, "type"=w1509) -> ("data"=w1513:i32)  [unwired: 1 in, 1 out]
        n163 = xnode "Database Variant To Data"("database variant"=w1531, "type"="") -> ("data"=w1525:string)  [unwired: 1 in, 1 out]
        n164 = Number To Decimal String(number=w1511) -> (decimal integer string=w1515:string)  [unwired: 1 in]
        n165 = Number To Decimal String(number=w1512) -> (decimal integer string=w1516:string)  [unwired: 1 in]
        n166 = Number To Decimal String(number=w1513) -> (decimal integer string=w1517:string)  [unwired: 1 in]
        n167 = Number To Decimal String(number=w1509) -> (decimal integer string=w1518:string)  [unwired: 1 in]
        n168 = Number To Decimal String(number=w1514) -> (decimal integer string=w1519:string)  [unwired: 1 in]
        n169 = Build Array(w1525, w1519, w1518, w1517, w1516, w1515, w1508) -> (w1524:string[])
        n170 = Insert Into Array(array=w1522, new element=w1524) -> (w1523:string[][])  [unwired: 2 in]
      }
      n171 = call <vilib>:"DB Tools Close Connection.vi"("error in (no error)"=w1498, "connection reference"=w1502) -> ("error out"=→"error out 4":errorcluster)  [unwired: 5 in]
      n172 = Add Array Elements(numeric array=w1480) -> (sum=w1475:i32)
      n173 = Add Array Elements(numeric array=w1479) -> (sum=w1474:i32)
      n174 = Add Array Elements(numeric array=w1481) -> (sum=w1476:i32)
      n175 = Add Array Elements(numeric array=w1478) -> (sum=w1473:i32)
      n176 = Add Array Elements(numeric array=w1477) -> (sum=w1472:i32)
      n177 = Add Array Elements(numeric array=w1459) -> (sum=w1460:i32)
      n178 = Number To Decimal String(number=w1472) -> (decimal integer string=w1466:string)  [unwired: 1 in]
      n179 = Number To Decimal String(number=w1476) -> (decimal integer string=w1470:string)  [unwired: 1 in]
      n180 = Number To Decimal String(number=w1475) -> (decimal integer string=w1469:string)  [unwired: 1 in]
      n181 = Number To Decimal String(number=w1474) -> (decimal integer string=w1468:string)  [unwired: 1 in]
      n182 = Number To Decimal String(number=w1473) -> (decimal integer string=w1467:string)  [unwired: 1 in]
      n183 = Number To Decimal String(number=w1460) -> (decimal integer string=w1458:string)  [unwired: 1 in]
      n184 = Build Array("", w1470, w1469, w1468, w1467, w1466, w1458) -> (w1463:string[])
      n185 = Insert Into Array(array=w1464, new element=w1463) -> (w1465:string[][])  [unwired: 2 in]
      n186 = local write "Table Control 3"(w1465) -> ()
    }
    frame #3 {
      w1785 = u16 1 items=["US", "Metric", "Default"] ("measurement system")
      w1786 = "M100DailyWIP"
      w1807 = T3."Excel"  # Report Type
      # "Simulate UUT Testing"
      # "Append Table to Report"
      # "Get Worksheet"
      n187 = call <vilib>:"New Report.vi"("report type"=w1807, "template (empty)"="Report Template") -> ("report out"=w1802:refnum<class "NI_report.lvclass">, "error out"=w1801:errorcluster)  [unwired: 12 in]
      n188 = call <vilib>:"Excel Get Worksheet.vi"("report in"=w1802, "worksheet index (0)"=0, "error in (no error)"=w1801) -> ("report out"=w1791:refnum<class "NI_report.lvclass">, "error out"=w1790:errorcluster)  [unwired: 11 in]
      n189 = Get Date/Time In Seconds() -> (seconds since 1Jan1904=w1756:timestamp)
      n190 = call-poly <vilib>:"Append Table to Report.vi"("report in"=w1791, "column width (1)"=1.5, "measurement system"=w1785, "column headers"=string[] ["Customer", "Package", "Incoming", "IQC", "Sorting", "DE", "MT", "RT", "EQC", "SLT", "CT1", "MK1", "DMHCL", "ExTray", "ExTrayE", "ExTube", "Baking", "LS", "LSVM", "LSTR", "TR", "TRVM", "VM", "Label", "FQC", "DP", "PK", "OQC", "WH", "Total"] ("row headers"), "text data"="Table Control", "error in (no error)"=w1790) -> ("report out"=w1804:refnum<class "NI_report.lvclass">, "error out"=w1803:errorcluster)  [unwired: 6 in, 2 out]
      n191 = Get Date/Time String(seconds (now)=w1756) -> (date string=w1758:string, time string=w1757:string)  [unwired: 2 in]
      n192 = call <vilib>:"Excel Insert Cells.vi"("report in"=w1804, "error in (no error)"=w1803) -> ("report out"=w1798:refnum<class "NI_report.lvclass">, "error out"=w1797:errorcluster)  [unwired: 12 in]
      n193 = Concatenate Strings("Report Time : " ("string"), w1758, " " ("string"), w1757) -> (w1794:string)
      n194 = call <vilib>:"Excel Easy Text.vi"("report in"=w1798, "text"=w1794, "start (-1, -1)"=cluster{"row":i32, "column":i32} {"row"=0, "column"=0} ("end (-1, -1)"), "error in (no error)"=w1797) -> ("report out"=w1779:refnum<class "NI_report.lvclass">, "error out"=w1778:errorcluster)  [unwired: 7 in, 3 out]
      n195 = call <vilib>:"Excel Get Worksheet.vi"("report in"=w1779, "worksheet index (0)"=1, "error in (no error)"=w1778) -> ("report out"=w1776:refnum<class "NI_report.lvclass">, "error out"=w1775:errorcluster)  [unwired: 11 in]
      n196 = call-poly <vilib>:"Append Table to Report.vi"("report in"=w1776, "column headers"=string[] ["Customer", "Package", "Product", "Status", "Qty", "Machine List"], "text data"="Table Control 2", "error in (no error)"=w1775) -> ("report out"=w1772:refnum<class "NI_report.lvclass">, "error out"=w1771:errorcluster)  [unwired: 8 in, 2 out]
      n197 = call <vilib>:"Excel Get Worksheet.vi"("report in"=w1772, "worksheet index (0)"=2, "error in (no error)"=w1771) -> ("report out"=w1770:refnum<class "NI_report.lvclass">, "error out"=w1769:errorcluster)  [unwired: 11 in]
      n198 = call-poly <vilib>:"Append Table to Report.vi"("report in"=w1770, "column headers"=string[] ["Customer", "RUN", "SETUP", "ENG", "IDLE", "OTHERS", "TOTAL"], "text data"="Table Control 3", "error in (no error)"=w1769) -> ("report out"=w1765:refnum<class "NI_report.lvclass">, "error out"=w1763:errorcluster)  [unwired: 8 in, 2 out]
      n199 = call <vilib>:"Excel Run Macro.vi"("report in"=w1765, "macro name"="macro1", "error in (no error)"=w1763) -> ("report out"=w1764:refnum<class "NI_report.lvclass">, "error out"=w1762:errorcluster)  [unwired: 10 in, 1 out]
      n200 = Format Date/Time String(time format string (%c)="%Y%m%d%H", seconds (now)=w1756) -> (date/time string=w1783:string)  [unwired: 1 in]
      n201 = Concatenate Strings(w1786, w1783, ".xls" ("string")) -> (w1787:string)
      n202 = Concatenate Strings(w1786, w1783) -> ()  [unwired: 1 out]
      n203 = Build Path(base path=path "o:/monitor/report", name or relative path=w1787) -> (appended path=w1781:path)
      n204 = call-dynamic "Save Report to File.vi"("report in"=w1764, "report file path"=w1781, "error in (no error)"=w1762) -> ("report out"=w1793:refnum<class "NI_report.lvclass">, "error out"=w1792:errorcluster)  [unwired: 11 in]
      n205 = call-dynamic "Dispose Report.vi"("report in"=w1793, "save changes? (F)"=FALSE, "error in (no error)"=w1792) -> ("error out"=→"error out 2":errorcluster)  [unwired: 12 in]
    }
    frame #4 {
      n206 = Index Array(array=w1810) -> (element=w1813:i32)  [unwired: 1 in]
      n207 = Greater?(x=w1813, y=1) -> (0:w1811:bool)
      n208 = case shown="True" w1811 {
        tunnel: w1809 -> [_ w1815]
        tunnel: w1808 -> [_ w1816]
        frame False {
        }
        frame True {
          (unwired) string[] ["yyliao@ptse.com.tw", "eric_fan@ptse.com.tw", "saulwang@ptse.com.tw"] ("recipients")
          n209 = Current VI's Path() -> (path=w1820:path)
          n210 = Strip Path(path=w1820) -> (name=w1819:string)  [unwired: 1 out]
          n211 = Match Pattern(string=w1819, regular expression=".vi") -> (before substring=w1817:string)  [unwired: 1 in, 3 out]
          n212 = call "MailMessage.vi"("AddSubject"=w1816, "message"="如附件", "file path"=w1815, "program"=w1817) -> ()  [unwired: 8 in]
        }
      }
    }
    frame #5 {
      n213 = Quit LabVIEW() -> ()  [unwired: 1 in]
    }
  }
